vi "sub_dt.vi"() -> (3 "dt":u32)   [LabVIEW 2018]
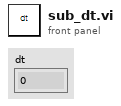
[diagram p1: front panel]
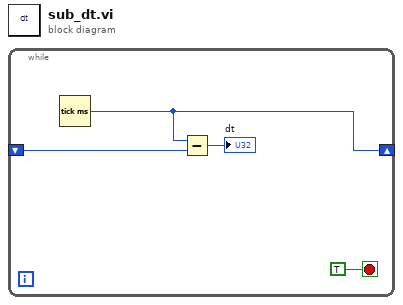
[diagram p0: block diagram]
diagram:
  n1 = while {
    shift-right: [w1] -> _
    shift-left: _ -> [w3]
    stop <- TRUE stop-if-true
    n2 = Tick Count (ms)() -> (millisecond timer value=w1:u32)
    n3 = Subtract(x=w1, y=w3) -> (x-y=→"dt":u32)
  }
